vi "Image Caption Cell.vi"(5 "Cell format":T2={"Font"={"Name"="Helvetica", "Size"=12.0, "Color"=0, "Style"={"Bold"=FALSE, "Italic"=FALSE, "Underline"=FALSE, "Strikeout"=FALSE}}, "Align. and LS"={"Horizontal"=enum."LEFT", "Vertical"=enum."BOTTOM", "Line spacing"=enum."1.0"}, "Border"={"Show?"=FALSE, "Thickness (point)"=0.0, "Color"=0}}, 6 "Aligment":string="JUSTIFY", 7 "String":string, 8 "error in (no error)":errorcluster, 9 "font":refnum<k24>, 10 "Leading":T1=18.0) -> (0 "error out":errorcluster, 2 "PdfP Cell":refnum<k24>)   [LabVIEW 2013]
doc: "Version 1.0\nDeveloped by Jean-Marc Simard\nCopyright © 2010, Exaprom Inc.\nAll rights reserved.\nLicense: BSD\n\nWith iTextSharp 4.1.6 (http://itextsharp.sourceforge.net)\nunder Mozilla Public License Version 1.1\n(http://www.mozilla.org/MPL/MPL-1.1.html)"
uses:
  C:/Users/MaxCorp/Documents/GitHub/TopView/DLL/itextsharp.dll
  DLL/itextsharp.dll
  <userlib>/Exaprom PDF/Controls/Cell Properties.ctl
  Controls/Font cluster.ctl
  Controls/Font size.ctl
  Controls/Font color.ctl
  Controls/Cell Vertical alignment.ctl
  Controls/Line spacing.ctl
  Controls/Image border.ctl
  Controls/Texte alignement.ctl
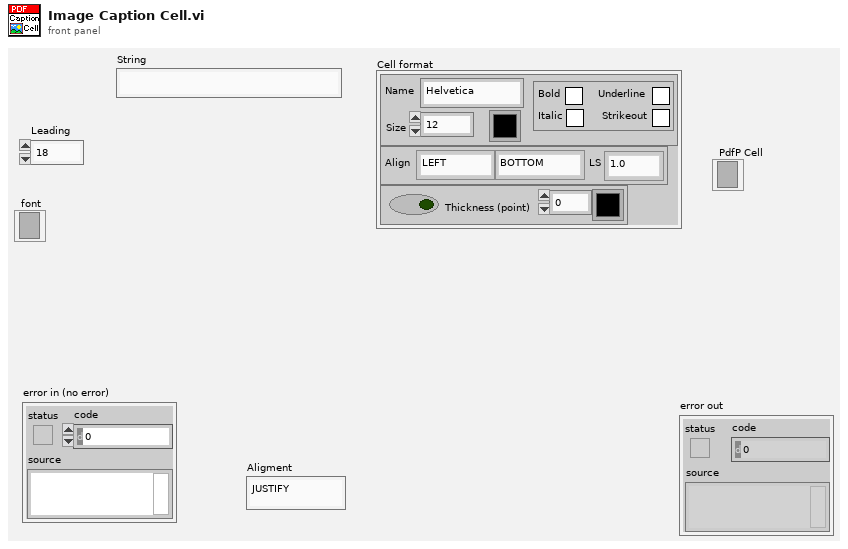
[diagram p1: front panel]
types:
  T1 = typedef "Font size.ctl" = sgl
  T2 = typedef "Cell Properties.ctl" = cluster{"Font":T3, "Align. and LS":cluster{"Horizontal":T5, "Vertical":T6, "Line spacing":T7}, "Border":T8}
  T3 = typedef "Font cluster.ctl" = cluster{"Name":string, "Size":T1, "Color":T4, "Style":cluster{"Bold":bool, "Italic":bool, "Underline":bool, "Strikeout":bool}}
  T4 = typedef "Font color.ctl" = u32
  T5 = typedef "Texte alignement.ctl" = enum16{"Select", "CENTER", "JUSTIFY", "LEFT", "RIGHT"}
  T6 = typedef "Cell Vertical alignment.ctl" = enum16{"TOP", "MIDDLE", "BOTTOM"}
  T7 = typedef "Line spacing.ctl" = enum16{"Select", "1.0", "1.5", "2.0"}
  T8 = typedef "Image border.ctl" = cluster{"Show?":bool, "Thickness (point)":sgl, "Color":u32}
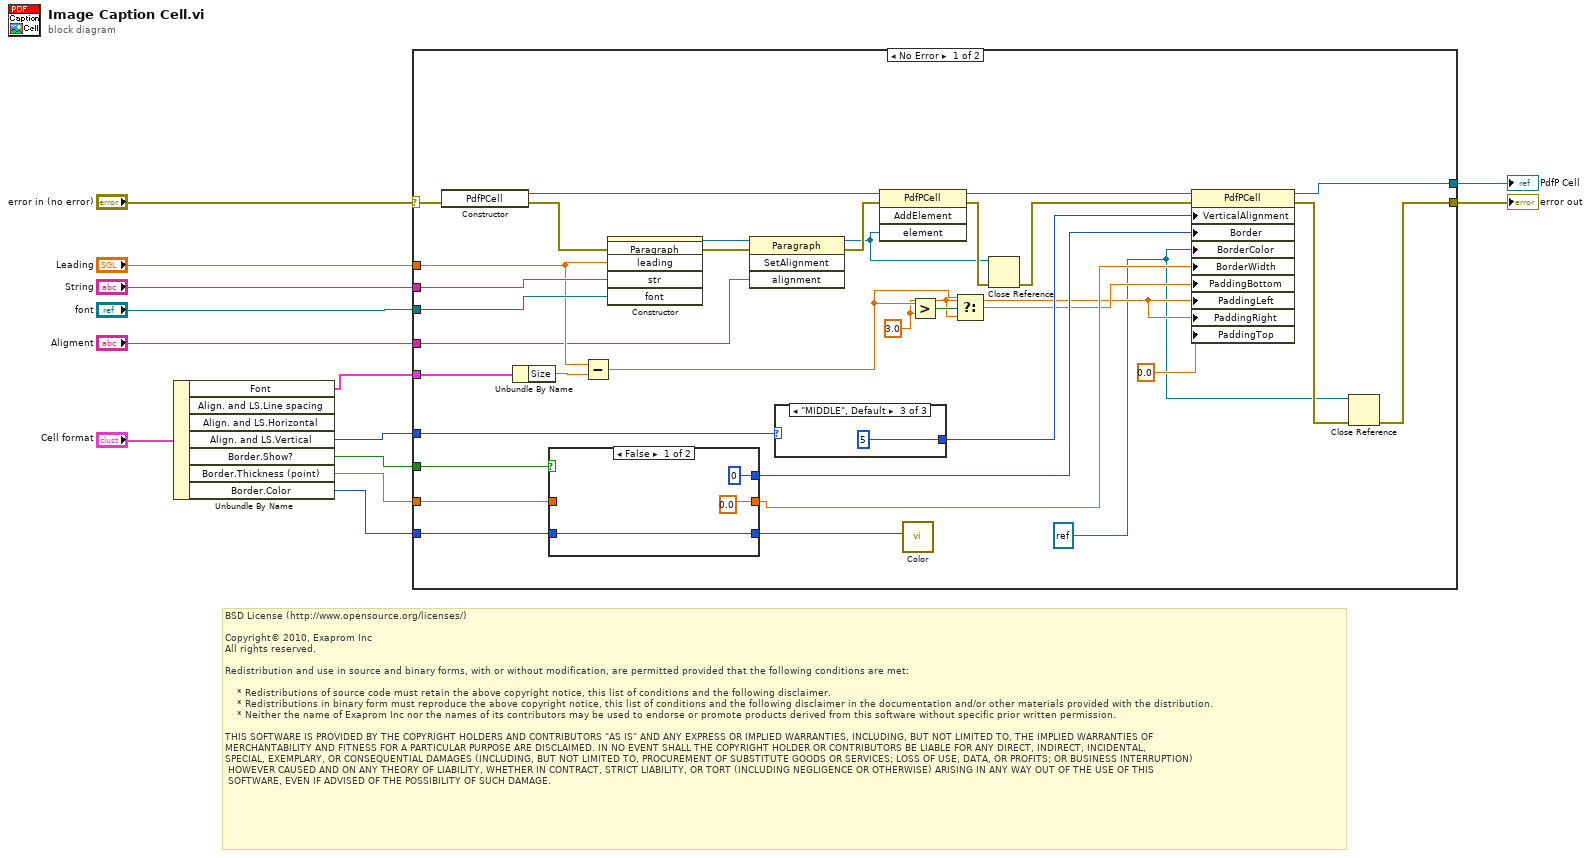
[diagram p0: block diagram]
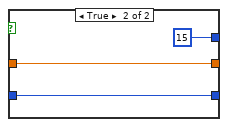
[diagram p2: hidden frame]
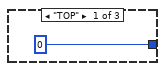
[diagram p3: hidden frame]
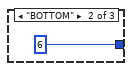
[diagram p4: hidden frame]
diagram:
  # "BSD License (http://www.opensource.org/licenses/)\n\nCopyright© 2010, Exaprom Inc\nAll rights reserved.\n\nRedistribution and use in source and binary forms, with or without modification, are permitted provided that the following conditions are met:\n\n    * Redistributions of source code must retain the above copyright notice, this list of conditions and the following disclaimer.\n    * Redistributions in binary form must reproduce the above copyright notice, this list of conditions and the following disclaimer in the documentation and/or other materials provided with the distribution.\n    * Neither the name of Exaprom Inc nor the names of its contributors may be used to endorse or promote products derived from this software without specific prior written permission.\n\nTHIS SOFTWARE IS PROVIDED BY THE COPYRIGHT HOLDERS AND CONTRIBUTORS \"AS IS\" AND ANY EXPRESS OR IMPLIED WARRANTIES, INCLUDING, BUT NOT LIMITED TO, THE IMPLIED WARRANTIES OF \nMERCHANTABILITY AND FITNESS FOR A PARTICULAR PURPOSE ARE DISCLAIMED. IN NO EVENT SHALL THE COPYRIGHT HOLDER OR CONTRIBUTORS BE LIABLE FOR ANY DIRECT, INDIRECT, INCIDENTAL,\nSPECIAL, EXEMPLARY, OR CONSEQUENTIAL DAMAGES (INCLUDING, BUT NOT LIMITED TO, PROCUREMENT OF SUBSTITUTE GOODS OR SERVICES; LOSS OF USE, DATA, OR PROFITS; OR BUSINESS INTERRUPTION)\n HOWEVER CAUSED AND ON ANY THEORY OF LIABILITY, WHETHER IN CONTRACT, STRICT LIABILITY, OR TORT (INCLUDING NEGLIGENCE OR OTHERWISE) ARISING IN ANY WAY OUT OF THE USE OF THIS\n SOFTWARE, EVEN IF ADVISED OF THE POSSIBILITY OF SUCH DAMAGE."
  n1 = Unbundle By Name("Cell format") -> ("Font"=w5:T3, "Align. and LS.Vertical"=w9:T6, "Border.Show?"=w8:bool, "Border.Thickness (point)"=w7:sgl, "Border.Color"=w6:u32)  [unwired: 2 out]
  n2 = case shown="No Error" "error in (no error)" {
    selector: "error in (no error)" -> [w42 w57]
    tunnel: [w15 w57] -> w12
    tunnel: w5 -> [w19 _]
    tunnel: "String" -> [w41 _]
    tunnel: w9 -> [w40 _]
    tunnel: w7 -> [w37 _]
    tunnel: w6 -> [w36 _]
    tunnel: w8 -> [w38 _]
    tunnel: "font" -> [w22 _]
    tunnel: "Leading" -> [w20 _]
    tunnel: "Aligment" -> [w18 _]
    tunnel: [w14 refnum<k24> refnum ("new reference")] -> w1
    frame No Error {
      w16 = refnum<k24> refnum ("BorderColor")
      w23 = sgl 3.0 ("t")
      n3 = constructor class="PdfPCell"(error in=w42) -> (reference out=w46:refnum<k24>, error out=w17:errorcluster)  [unwired: 2 in, 1 out]
      n4 = Unbundle By Name(w19) -> ("Size"=w33:T1)
      n5 = case shown="False" w38 {
        tunnel: [sgl 0.0 ("BorderWidth") w51] -> w34
        tunnel: w37 -> [_ w51]
        tunnel: [w48 w50] -> w27
        tunnel: w36 -> [w48 w50]
        tunnel: [0 15] -> w35
        frame False {
        }
        frame True {
        }
      }
      n6 = Subtract(x=w20, y=w33) -> (x-y=w25:T1)
      n7 = constructor class="Paragraph"(error in=w17, "leading"=w20, "str"=w41, "font"=w22) -> (reference out=w45:refnum<k24>, error out=w21:errorcluster)  [unwired: 2 in, 4 out]
      n8 = invoke class="Paragraph" method="SetAlignment"(reference=w45, error in=w21, "alignment"=w18) -> (reference out=w30:refnum<k24>, error out=w44:errorcluster)  [unwired: 1 in, 2 out]
      n9 = case shown="\"MIDDLE\", Default" w40 {
        tunnel: [0 6 5] -> w39
        frame "TOP" {
        }
        frame "BOTTOM" {
        }
        frame "MIDDLE", Default {
        }
      }
      n10 = invoke class="PdfPCell" method="AddElement"(reference=w46, error in=w44, "element"=w30) -> (reference out=w43:refnum<k24>, error out=w31:errorcluster)  [unwired: 1 in, 2 out]
      n11 = call "Color.vi"("Color"=w27) -> ()  [unwired: 1 in, 10 out]
      n12 = Greater?(x=w25, y=w23) -> (0:w26:bool)
      n13 = Select(t=w25, s=w26, f=w23) -> (s? t:f=w24:T1)
      n14 = Close Reference(reference=w30, error in (no error)=w31) -> (error out=w28:errorcluster)
      n15 = property class="PdfPCell"(reference=w43, error in=w28, "VerticalAlignment"=w39, "Border"=w35, "BorderColor"=w16, "BorderWidth"=w34, "PaddingBottom"=w24, "PaddingLeft"=w23, "PaddingRight"=w23, "PaddingTop"=sgl 0.0) -> (reference out=w14:refnum<k24>, error out=w29:errorcluster)
      n16 = Close Reference(reference=w16, error in (no error)=w29) -> (error out=w15:errorcluster)
    }
    frame Error {
    }
  }
  "error out" <- w12
  "PdfP Cell" <- w1
